vi "Exec FPGA.vi"() -> ()   [LabVIEW 2023]
uses:
  <vilib>/LabVIEW Targets/FPGA/cRIO/shared/nicrio_ModuleControls/nicrio_cRIO-9467_Latitude.ctl
  <vilib>/LabVIEW Targets/FPGA/cRIO/shared/nicrio_ModuleControls/nicrio_cRIO-9467_Longitude.ctl
  <vilib>/LabVIEW Targets/FPGA/cRIO/shared/nicrio_ModuleControls/nicrio_cRIO-9467_Altitude.ctl
  <vilib>/rvi/Emulation/niFpgaGetClockAttributes.vi
  <vilib>/rvi/Emulation/niFpgaSctlEmulationGetInTimedLoop.vi
  <vilib>/rvi/Emulation/niFpgaEmulationReportErrorSimple.vi
  subVIs/Front Panel Globals.vi
  <vilib>/rvi/Emulation/niFpgaProcessEmulError.vi
  <vilib>/rvi/Emulation/niFpgaCriticalErrorInLSC.vi
  <vilib>/rvi/DataTransferAndStorage/Container/XNode/niFpgaContainer.xnode
  <vilib>/rvi/interface/RandomDataEmulation/nirviRandomDataFpgaReadWriteTemplate.vi
panel:
  in  "PPS Count Ticks":u32=4000000
  out "PPS Trigger":bool
  out "GPS Time (nanoseconds)":u64
  out "GPS Time (seconds)":u64
  out "Analog Channel Count":i32
  in  "Enable Analog Acquisition":bool
  out "Analog Acquisition Looprate":sgl
  in  "Analog Acquisition Rate":sgl=10000.0
  in  "Watchdog Whack":bool
  out "GPS Self-Survey Complete":bool
  out "GPS Firmware Version":u32
  out "GPS Vendor ID":u16
  out "GPS Altitude (m)":T1 format="%.2f"
  out "GPS Longitude (°)":T2 format="%.6g"
  out "GPS Latitude (°)":T3 format="%.6f"
  out "GPS Serial Number":u32
  out "GPS Time Lock":bool
  out "GPS Time (ns)":u64
  out "GPS Status":T4(ring)
  out "GPS Time Offset":i32
  out "GPS Antenna Status":T5(ring)
  out "GPS Satelites Available":u8
  out "GPS UTC Offset":i8
  out "GPS UTC Offset Valid":bool
  in  "FPGA USER1 LED":bool
  out "Watchdog Whack Count":u32
  in  "System Reset":bool
  out "Watchdog ms Since Whack":u32
  in  "Watchdog Timeout (ms)":u32=3600000
  in  "Watchdog Enable":bool
  out "FPGA Nanosecond Counter":i64
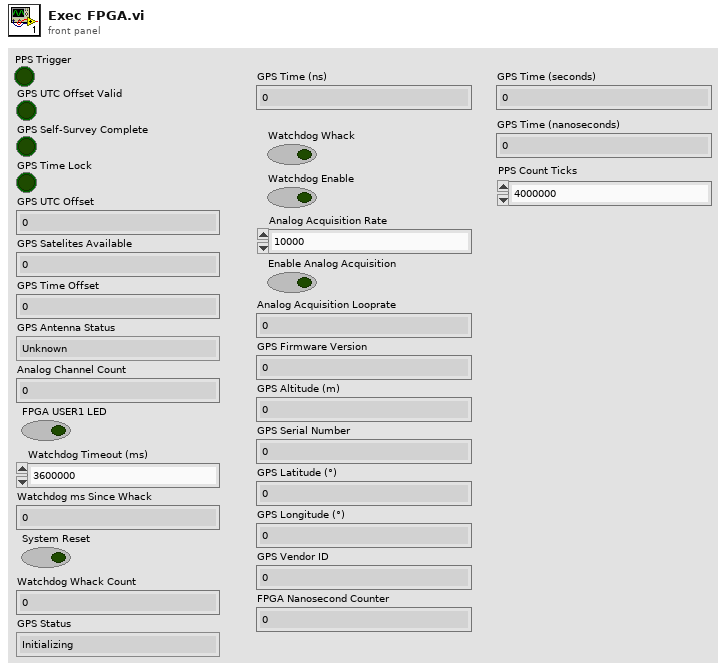
[diagram p1: front panel]
types:
  T1 = typedef "nicrio_cRIO-9467_Altitude.ctl" = fxp<+/-,24,17>
  T2 = typedef "nicrio_cRIO-9467_Longitude.ctl" = fxp<+/-,29,9>
  T3 = typedef "nicrio_cRIO-9467_Latitude.ctl" = fxp<+/-,28,8>
  T4 = enum8{"Initializing", "Normal", "Unable to get fix"}
  T5 = enum8{"Unknown", "Normal", "Absent", "Overcurrent"}
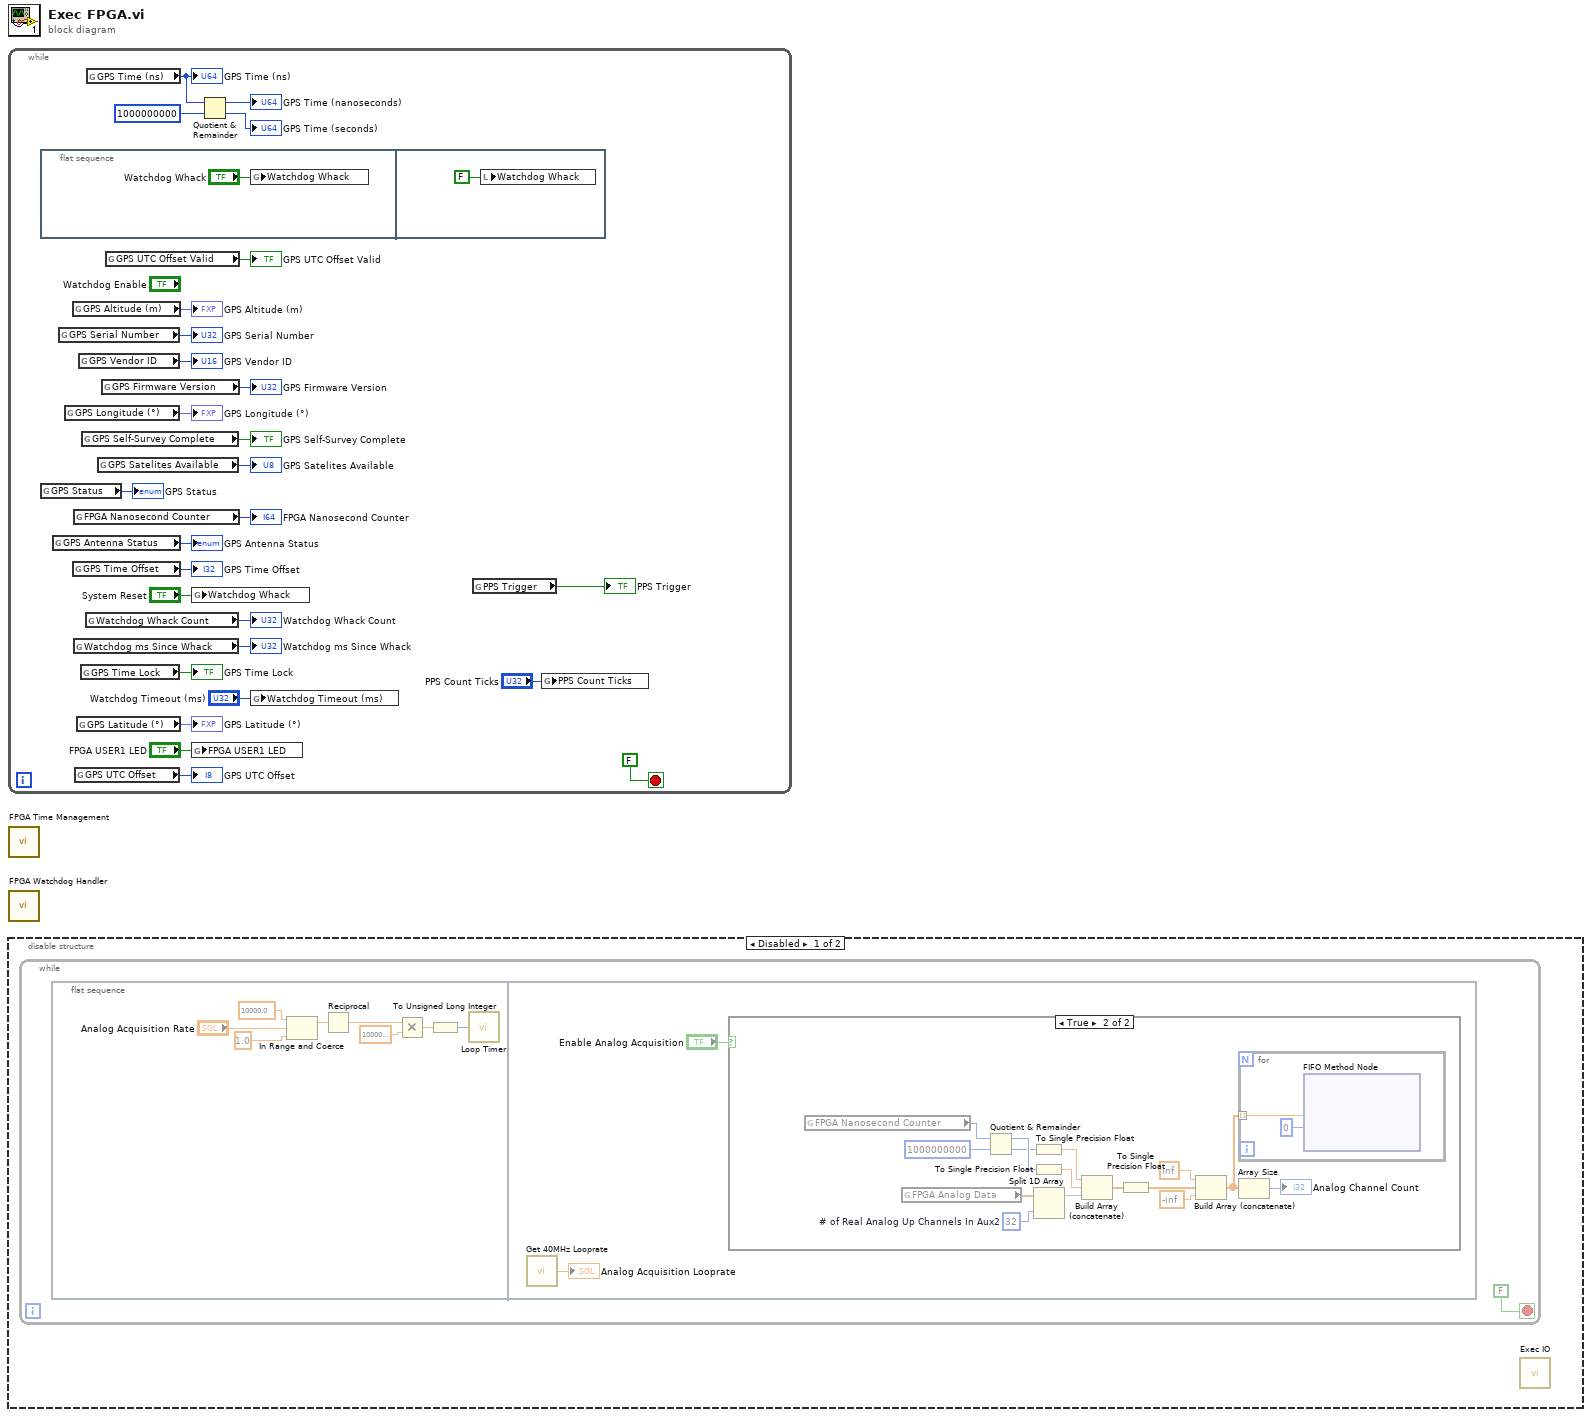
[diagram p0: block diagram]
diagram:
  n1 = while {
    stop <- FALSE stop-if-true
    n2 = flat-sequence {
      frame #0 {
        n3 = global write "Front Panel Globals.vi" "Watchdog Whack"("Watchdog Whack") -> ()
      }
      frame #1 {
        n4 = local write "Watchdog Whack"(FALSE ("Watchdog Enable")) -> ()
      }
    }
    n5 = global read "Front Panel Globals.vi" "GPS Status"() -> (→"GPS Status":T4)
    n6 = global read "Front Panel Globals.vi" "GPS Antenna Status"() -> (→"GPS Antenna Status":T5)
    n7 = global read "Front Panel Globals.vi" "GPS Serial Number"() -> (→"GPS Serial Number":u32)
    n8 = global read "Front Panel Globals.vi" "GPS Longitude (°)"() -> (→"GPS Longitude (°)":T2)
    n9 = global read "Front Panel Globals.vi" "GPS Altitude (m)"() -> (→"GPS Altitude (m)":T1)
    n10 = global read "Front Panel Globals.vi" "GPS Time Offset"() -> (→"GPS Time Offset":i32)
    n11 = global read "Front Panel Globals.vi" "FPGA Nanosecond Counter"() -> (→"FPGA Nanosecond Counter":i64)
    n12 = global read "Front Panel Globals.vi" "Watchdog ms Since Whack"() -> (→"Watchdog ms Since Whack":u32)
    n13 = global read "Front Panel Globals.vi" "GPS UTC Offset"() -> (→"GPS UTC Offset":i8)
    n14 = global read "Front Panel Globals.vi" "GPS Latitude (°)"() -> (→"GPS Latitude (°)":T3)
    n15 = global read "Front Panel Globals.vi" "GPS Vendor ID"() -> (→"GPS Vendor ID":u16)
    n16 = global read "Front Panel Globals.vi" "GPS Time Lock"() -> (→"GPS Time Lock":bool)
    n17 = global read "Front Panel Globals.vi" "GPS Self-Survey Complete"() -> (→"GPS Self-Survey Complete":bool)
    n18 = global read "Front Panel Globals.vi" "Watchdog Whack Count"() -> (→"Watchdog Whack Count":u32)
    n19 = global read "Front Panel Globals.vi" "GPS Time (ns)"() -> (w6:u64)
    "GPS Time (ns)" <- w6
    n20 = global read "Front Panel Globals.vi" "GPS Satelites Available"() -> (→"GPS Satelites Available":u8)
    n21 = global read "Front Panel Globals.vi" "GPS Firmware Version"() -> (→"GPS Firmware Version":u32)
    n22 = global read "Front Panel Globals.vi" "GPS UTC Offset Valid"() -> (→"GPS UTC Offset Valid":bool)
    n23 = global write "Front Panel Globals.vi" "Watchdog Whack"("System Reset") -> ()
    n24 = global write "Front Panel Globals.vi" "FPGA USER1 LED"("FPGA USER1 LED") -> ()
    n25 = Quotient & Remainder(x=w6, y=u64 1000000000) -> (x-y*floor(x/y)=→"GPS Time (nanoseconds)":u64, floor(x/y)=→"GPS Time (seconds)":u64)
    n26 = global write "Front Panel Globals.vi" "Watchdog Timeout (ms)"("Watchdog Timeout (ms)") -> ()
    n27 = global read "Front Panel Globals.vi" "PPS Trigger"() -> (→"PPS Trigger":bool)
    n28 = global write "Front Panel Globals.vi" "PPS Count Ticks"("PPS Count Ticks") -> ()
  }
  n29 = call "FPGA Time Management.vi"() -> ()  [unwired: 12 in]
  n30 = call "FPGA Watchdog Handler.vi"() -> ()  [unwired: 12 in]
  n31 = disable-structure shown="Disabled" {
    frame Disabled {
      n32 = while {
        stop <- FALSE stop-if-true
        n33 = flat-sequence {
          frame #0 {
            n34 = In Range and Coerce(upper limit=sgl 10000.0, x="Analog Acquisition Rate", lower limit=sgl 1.0) -> (coerced(x)=w35:sgl)  [unwired: 1 out]
            n35 = Reciprocal(x=w35) -> (1/x=w36:sgl)
            n36 = Multiply(x=w36, y=sgl 1000000.0 ("upper limit")) -> (x*y=w37:sgl)
            n37 = To Unsigned Long Integer(number=w37) -> (unsigned 32bit integer=w38:u32)
            n38 = call "Loop Timer"("Count(uSec)"=w38) -> ()  [unwired: 1 out]
          }
          frame #1 {
            n39 = call "Get 40MHz Looprate.vi"() -> ("Looprate"=→"Analog Acquisition Looprate":sgl)  [unwired: 5 in]
            n40 = case shown="True" "Enable Analog Acquisition" {
              frame False {
              }
              frame True {
                w41 = 32  # # of Real Analog Up Channels In Aux2
                n41 = global read "Front Panel Globals.vi" "FPGA Nanosecond Counter"() -> (w48:i64)
                n42 = global read "Front Panel Globals.vi" "FPGA Analog Data"() -> (w44:sgl[])
                n43 = Quotient & Remainder(x=w48, y=i64 1000000000) -> (x-y*floor(x/y)=w51:i64, floor(x/y)=w50:i64)
                n44 = To Single Precision Float(number=w50) -> (single precision float=w46:sgl)
                n45 = To Single Precision Float(number=w51) -> (single precision float=w45:sgl)
                n46 = Split 1D Array(array=w44, index=w41) -> (first subarray=w43:sgl[])  [unwired: 1 out]
                n47 = Build Array (concatenate)(w46, w45, w43) -> (w53:sgl[])
                n48 = To Single Precision Float(number=w53) -> (single precision float=w47:sgl[])
                n49 = Build Array (concatenate)(sgl inf ("Mod1/CH3"), w47, sgl -inf ("Mod1/CH3")) -> (w42:sgl[])
                n50 = for {
                  tunnel: w42 -> [w57] mode=indexing
                  n51 = xnode ("FIFO Method Node")("Element"=w57, "Timeout"=0) -> ()  [unwired: 1 in, 2 out]
                }
                n52 = Array Size(array=w42) -> (size(s)=→"Analog Channel Count":i32)
              }
            }
          }
        }
      }
      n53 = call "Exec IO.vi"() -> ()  [unwired: 12 in]
    }
    frame Enabled {
    }
  }
